vi "Radau5_Update RK Data.vi"(11 "Implicit RK Data In":T1) -> (3 "Implicit RK Data Out":T1)   [LabVIEW 2020, in "NI_DAE.lvlib"]
uses:
  <vilib>/gmath/NI_DAE.lvlib
  <vilib>/gmath/dae.llb/Radau5_Implicit RK Data.ctl
  <vilib>/gmath/dae.llb/Radau5_RK Status.ctl
  <vilib>/Analysis/Matrix/Datatypes/RealMatrix.ctl
  <vilib>/Analysis/Matrix/Datatypes/ComplexMatrix.ctl
  <vilib>/Analysis/Matrix/NI_Matrix.lvlib
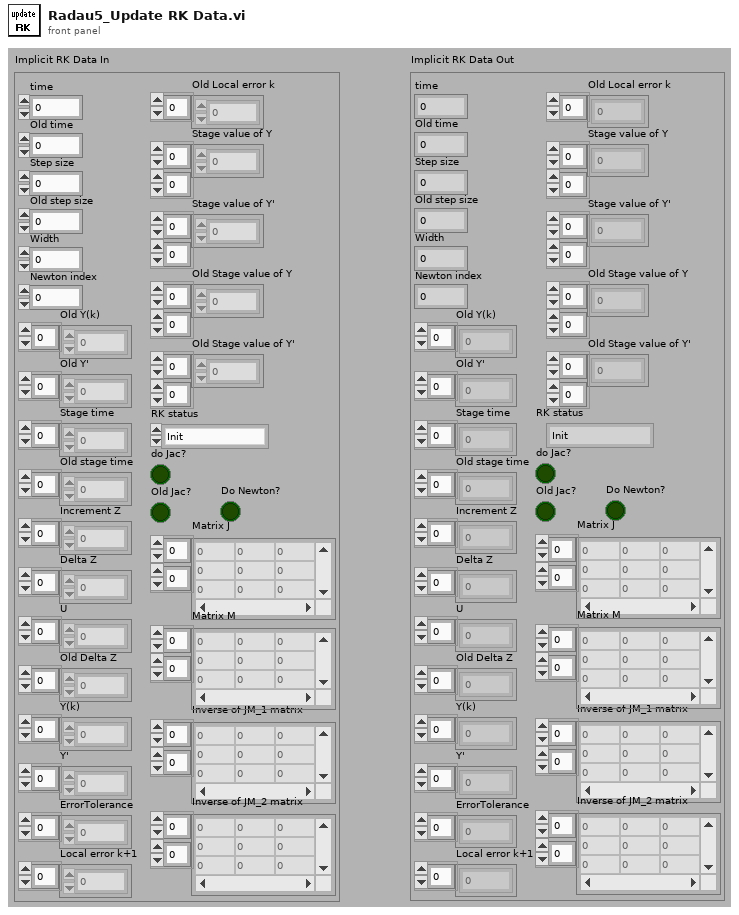
[diagram p1: front panel]
types:
  T1 = typedef "NI_DAE.lvlib/Radau5_Implicit RK Data.ctl" = cluster{"time":dbl, "Old time":dbl, "Step size":dbl, "Old step size":dbl, "Width":i32, "Newton index":i32, "Old Y(k)":dbl[], "Old Y'":dbl[], "Stage time":dbl[], "Old stage time":dbl[], "Increment Z":dbl[], "Delta Z":dbl[], "U":dbl[], "Old Delta Z":dbl[], "Y(k)":dbl[], "Y'":dbl[], "ErrorTolerance":dbl[], "Local error k+1":dbl[], "Old Local error k":dbl[], "Stage value of Y":dbl[][], "Stage value of Y'":dbl[][], "Old Stage value of Y":dbl[][], "Old Stage value of Y'":dbl[][], "RK status":T2, "do Jac?":bool, "Old Jac?":bool, "Do Newton?":bool, "Matrix J":T3, "Matrix M":T3, "Inverse of JM_1 matrix ":T3, "Inverse of JM_2 matrix":T4}
  T2 = typedef "NI_DAE.lvlib/Radau5_RK Status.ctl" = enum16{"Init", "Predict", "Jacobian", "Newton", "error eval y y'", "error eval calc", "next step updata", "reset RK"}
  T3 = typedef "NI_Matrix.lvlib/RealMatrix.ctl" = dbl[][]
  T4 = typedef "NI_Matrix.lvlib/ComplexMatrix.ctl" = cdb[][]
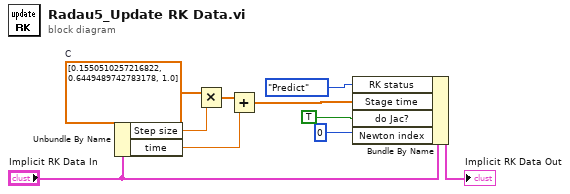
[diagram p0: block diagram]
diagram:
  w9 = dbl[] [0.1550510257216822, 0.6449489742783178, 1.0]  # C
  n1 = Unbundle By Name("Implicit RK Data In") -> ("Step size"=w8:dbl, "time"=w6:dbl)
  n2 = Multiply(x=w9, y=w8) -> (x*y=w7:dbl[])
  n3 = Add(x=w7, y=w6) -> (x+y=w5:dbl[])
  n4 = Bundle By Name(cluster="Implicit RK Data In", "RK status"=Radau5_RK_Status."Predict", "Stage time"=w5, "do Jac?"=TRUE, "Newton index"=0) -> (→"Implicit RK Data Out":T1)
